vi "Clear All Memory Blocks.vi"   [LabVIEW 2016, in "CVT.lvlib" / "Current Value Table.lvlib"]
doc: "This clears all memory blocks. New data types should be added to this VI."
uses:
  <vilib>/NI/Current Value Table/Current Value Table.lvlib
  <vilib>/NI/Current Value Table/Type Defs/Memory Commands.ctl
  <vilib>/NI/Current Value Table/DataTypes/Double_Memory Block.vi
  <vilib>/NI/Current Value Table/DataTypes/Single_Memory Block.vi
  <vilib>/NI/Current Value Table/DataTypes/I64_Memory Block.vi
  <vilib>/NI/Current Value Table/DataTypes/I32_Memory Block.vi
  <vilib>/NI/Current Value Table/DataTypes/I16_Memory Block.vi
  <vilib>/NI/Current Value Table/DataTypes/I8_Memory Block.vi
  <vilib>/NI/Current Value Table/DataTypes/U64_Memory Block.vi
  <vilib>/NI/Current Value Table/DataTypes/U32_Memory Block.vi
  <vilib>/NI/Current Value Table/DataTypes/U16_Memory Block.vi
  <vilib>/NI/Current Value Table/DataTypes/U8_Memory Block.vi
  <vilib>/NI/Current Value Table/DataTypes/String_Memory Block.vi
  <vilib>/NI/Current Value Table/DataTypes/Boolean_Memory Block.vi
  <vilib>/NI/Current Value Table/DataTypes/Array of U8_Memory Block.vi
  <vilib>/NI/Current Value Table/DataTypes/Array of U16_Memory Block.vi
  <vilib>/NI/Current Value Table/DataTypes/Array of U32_Memory Block.vi
  <vilib>/NI/Current Value Table/DataTypes/Array of U64_Memory Block.vi
  <vilib>/NI/Current Value Table/DataTypes/Array of I64_Memory Block.vi
  <vilib>/NI/Current Value Table/DataTypes/Array of I32_Memory Block.vi
  <vilib>/NI/Current Value Table/DataTypes/Array of I16_Memory Block.vi
  <vilib>/NI/Current Value Table/DataTypes/Array of I8_Memory Block.vi
  <vilib>/NI/Current Value Table/DataTypes/Array of Double_Memory Block.vi
  <vilib>/NI/Current Value Table/DataTypes/Array of Single_Memory Block.vi
  <vilib>/NI/Current Value Table/DataTypes/Array of Boolean_Memory Block.vi
  <vilib>/NI/Current Value Table/DataTypes/Array of String_Memory Block.vi
types:
  T1 = typedef "CVT.lvlib/Current Value Table.lvlib/Memory Commands.ctl" = enum16{"Init", "Add Data", "Read", "Read Group", "Read All", "Write", "Write Group", "Get Size"}
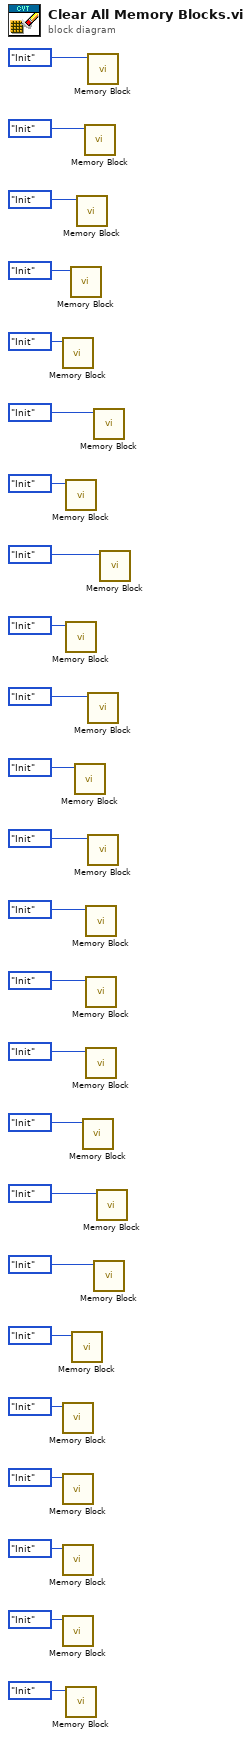
[diagram p0: block diagram]
diagram:
  n1 = call-poly <vilib>:"Memory Block.vi"("Method"=Memory_Commands."Init") -> ()  [unwired: 8 in, 3 out]
  n2 = call-poly <vilib>:"Memory Block.vi"("Method"=Memory_Commands."Init") -> ()  [unwired: 8 in, 3 out]
  n3 = call-poly <vilib>:"Memory Block.vi"("Method"=Memory_Commands."Init") -> ()  [unwired: 8 in, 3 out]
  n4 = call-poly <vilib>:"Memory Block.vi"("Method"=Memory_Commands."Init") -> ()  [unwired: 8 in, 3 out]
  n5 = call-poly <vilib>:"Memory Block.vi"("Method"=Memory_Commands."Init") -> ()  [unwired: 8 in, 3 out]
  n6 = call-poly <vilib>:"Memory Block.vi"("Method"=Memory_Commands."Init") -> ()  [unwired: 8 in, 3 out]
  n7 = call-poly <vilib>:"Memory Block.vi"("Method"=Memory_Commands."Init") -> ()  [unwired: 8 in, 3 out]
  n8 = call-poly <vilib>:"Memory Block.vi"("Method"=Memory_Commands."Init") -> ()  [unwired: 8 in, 3 out]
  n9 = call-poly <vilib>:"Memory Block.vi"("Method"=Memory_Commands."Init") -> ()  [unwired: 8 in, 3 out]
  n10 = call-poly <vilib>:"Memory Block.vi"("Method"=Memory_Commands."Init") -> ()  [unwired: 8 in, 3 out]
  n11 = call-poly <vilib>:"Memory Block.vi"("Method"=Memory_Commands."Init") -> ()  [unwired: 8 in, 3 out]
  n12 = call-poly <vilib>:"Memory Block.vi"("Method"=Memory_Commands."Init") -> ()  [unwired: 8 in, 3 out]
  n13 = call-poly <vilib>:"Memory Block.vi"("Method"=Memory_Commands."Init") -> ()  [unwired: 8 in, 3 out]
  n14 = call-poly <vilib>:"Memory Block.vi"("Method"=Memory_Commands."Init") -> ()  [unwired: 8 in, 3 out]
  n15 = call-poly <vilib>:"Memory Block.vi"("Method"=Memory_Commands."Init") -> ()  [unwired: 8 in, 3 out]
  n16 = call-poly <vilib>:"Memory Block.vi"("Method"=Memory_Commands."Init") -> ()  [unwired: 8 in, 3 out]
  n17 = call-poly <vilib>:"Memory Block.vi"("Method"=Memory_Commands."Init") -> ()  [unwired: 8 in, 3 out]
  n18 = call-poly <vilib>:"Memory Block.vi"("Method"=Memory_Commands."Init") -> ()  [unwired: 8 in, 3 out]
  n19 = call-poly <vilib>:"Memory Block.vi"("Method"=Memory_Commands."Init") -> ()  [unwired: 8 in, 3 out]
  n20 = call-poly <vilib>:"Memory Block.vi"("Method"=Memory_Commands."Init") -> ()  [unwired: 8 in, 3 out]
  n21 = call-poly <vilib>:"Memory Block.vi"("Method"=Memory_Commands."Init") -> ()  [unwired: 8 in, 3 out]
  n22 = call-poly <vilib>:"Memory Block.vi"("Method"=Memory_Commands."Init") -> ()  [unwired: 8 in, 3 out]
  n23 = call-poly <vilib>:"Memory Block.vi"("Method"=Memory_Commands."Init") -> ()  [unwired: 8 in, 3 out]
  n24 = call-poly <vilib>:"Memory Block.vi"("Method"=Memory_Commands."Init") -> ()  [unwired: 8 in, 3 out]
